vi "Offset Widget Actions 2 Transactions.vi"(9 "Number of LBCBs":T5, 11 "Offset Widget Actions":T6) -> (2 "Transactions":T1[](array[typedef]))   [LabVIEW 2009]
uses:
  Offset Widget Actions.ctl
  Data Access Objects/Application/Number Of LBCBs.ctl
  Global Data/Dataset Transaction Id.ctl
  Global Data/Dataset Source.ctl
  Global Data/Dataset Type.ctl
  Apps/Yes No Button.ctl
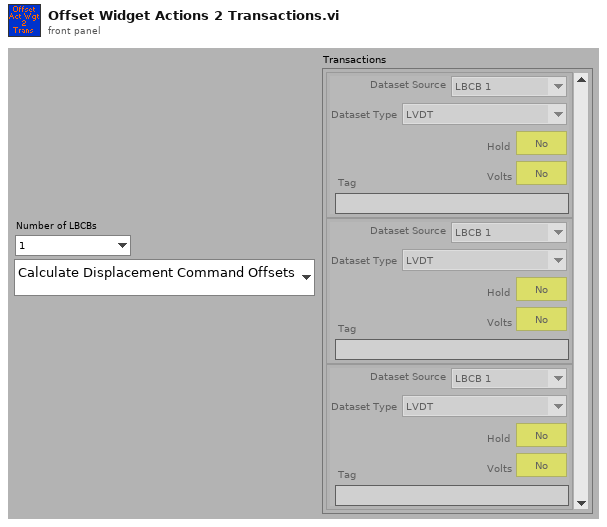
[diagram p1: front panel]
types:
  T1 = typedef "Dataset Transaction Id.ctl" = cluster{"Dataset Source":T2, "Dataset Type":T3, "Hold":T4, "Volts":T4, "Tag":string}
  T2 = typedef "Dataset Source.ctl" = enum16{"LBCB 1", "LBCB 2", "Combined", "External Sensors"}
  T3 = typedef "Dataset Type.ctl" = enum16{"LVDT", "Load Cell", "Actuator Command", "Servo Error", "Displacement Command", "Displacement", "Force"}
  T4 = typedef "Yes No Button.ctl" = bool
  T5 = typedef "Number Of LBCBs.ctl" = enum16{"1", "2"}
  T6 = typedef "Offset Widget Actions.ctl" = enum16{"Calculate Displacement Command Offsets", "Calculate Displacement Offsets", "Re-Calculate Force Offsets", "Calculate New Force Offsets", "Delete Force Offsets", "Calculate External Sensor Offsets"}
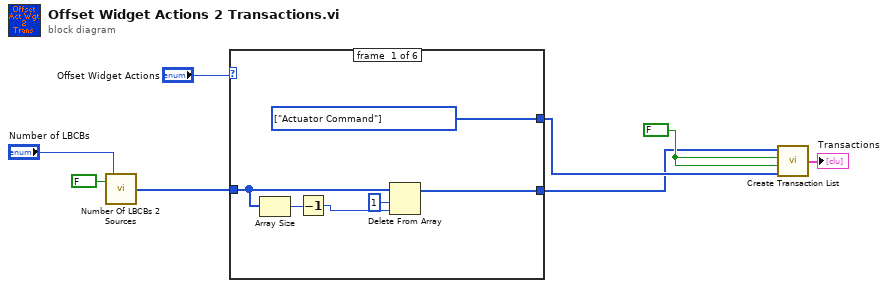
[diagram p0: block diagram]
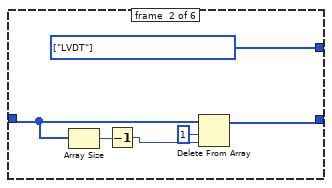
[diagram p2: hidden frame]
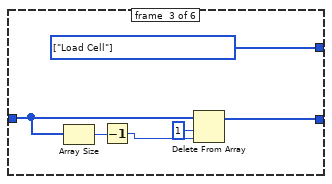
[diagram p3: hidden frame]
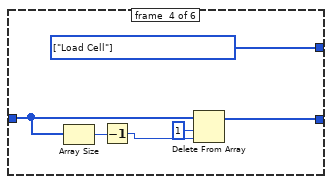
[diagram p4: hidden frame]
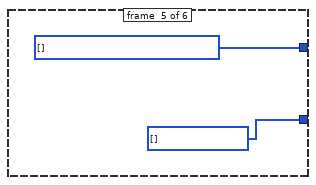
[diagram p5: hidden frame]
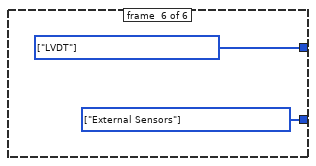
[diagram p6: hidden frame]
diagram:
  w5 = FALSE ("Include Volts")
  n1 = call "Number Of LBCBs 2 Sources.vi"("Number of LBCBs"="Number of LBCBs", "Combined LBCBs"=FALSE) -> ("Sources"=w4:T2[])
  n2 = case shown="\"Delete Force Offsets\"" "Offset Widget Actions" {
    tunnel: [w14 w20 w26 w32 w34 w36] -> w6
    tunnel: w4 -> [w13 w16 w21 w27 _ _]
    tunnel: [w9 w15 w22 w28 w33 w35] -> w3
    frame #0 {
      w14 = T3[] [enum."Actuator Command"] items=["LVDT", "Load Cell", "Actuator Command", "Servo Error", "Displacement Command", "Displacement", "Force"] ("Types")
      n3 = Array Size(array=w13) -> (size(s)=w12:i32)
      n4 = Decrement(x=w12) -> (x-1=w11:i32)
      n5 = Delete From Array(array=w13, length=1, index=w11) -> (array with subset deleted=w9:T2[])  [unwired: 1 out]
    }
    frame #1 {
      w20 = T3[] [enum."LVDT"] items=["LVDT", "Load Cell", "Actuator Command", "Servo Error", "Displacement Command", "Displacement", "Force"] ("Types")
      n6 = Array Size(array=w16) -> (size(s)=w17:i32)
      n7 = Decrement(x=w17) -> (x-1=w18:i32)
      n8 = Delete From Array(array=w16, length=1, index=w18) -> (array with subset deleted=w15:T2[])  [unwired: 1 out]
    }
    frame #2 {
      w26 = T3[] [enum."Load Cell"] items=["LVDT", "Load Cell", "Actuator Command", "Servo Error", "Displacement Command", "Displacement", "Force"] ("Types")
      n9 = Array Size(array=w21) -> (size(s)=w25:i32)
      n10 = Decrement(x=w25) -> (x-1=w24:i32)
      n11 = Delete From Array(array=w21, length=1, index=w24) -> (array with subset deleted=w22:T2[])  [unwired: 1 out]
    }
    frame #3 {
      w32 = T3[] [enum."Load Cell"] items=["LVDT", "Load Cell", "Actuator Command", "Servo Error", "Displacement Command", "Displacement", "Force"] ("Types")
      n12 = Array Size(array=w27) -> (size(s)=w31:i32)
      n13 = Decrement(x=w31) -> (x-1=w30:i32)
      n14 = Delete From Array(array=w27, length=1, index=w30) -> (array with subset deleted=w28:T2[])  [unwired: 1 out]
    }
    frame #4 {
      w33 = T2[] [] items=["LBCB 1", "LBCB 2", "Combined", "External Sensors"] ("Sources")
      w34 = T3[] [] items=["LVDT", "Load Cell", "Actuator Command", "Servo Error", "Displacement Command", "Displacement", "Force"] ("Types")
    }
    frame #5 {
      w35 = T2[] [enum."External Sensors"] items=["LBCB 1", "LBCB 2", "Combined", "External Sensors"] ("Sources")
      w36 = T3[] [enum."LVDT"] items=["LVDT", "Load Cell", "Actuator Command", "Servo Error", "Displacement Command", "Displacement", "Force"] ("Types")
    }
  }
  n15 = call "Create Transaction List.vi"("Types"=w6, "Hold"=w5, "Volts"=w5, "Sources"=w3) -> ("Transactions"=→"Transactions":T1[])
